vi "Read Coils.vi"(8 "error in (no error)":errorcluster, 9 "quantity":u16, 10 "starting address":u16, 11 "MB session in":refnum<class "MB_Master.lvclass">) -> (0 "error out":errorcluster, 2 "Coils":bool[](array[boolean]), 3 "MB session out":refnum<class "MB_Master.lvclass">)   [LabVIEW 2021, in "MB Master.lvlib"]
doc: "Function Code 1: Reads <b>quantity</b> number of coils starting from <b>starting address</b>"
uses:
  <vilib>/Plasmionique/MB Master/MB Master.lvlib
  <vilib>/Plasmionique/MB Master/MB_Master/MB_Master.lvclass
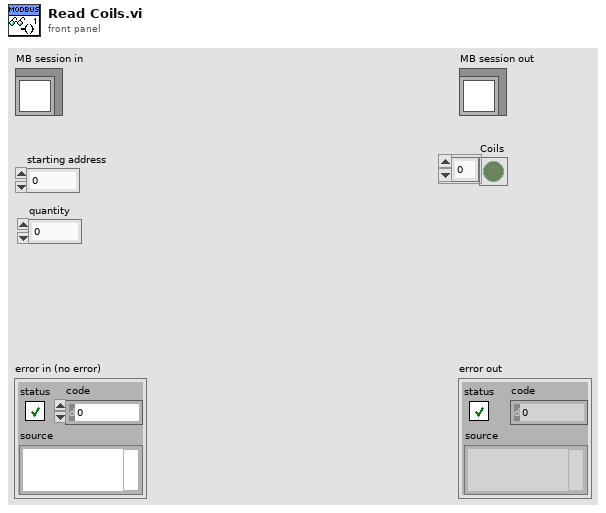
[diagram p1: front panel]
types:
  T1 = typedef "MB Master.lvlib/MB_PDU_Cluster.ctl" = cluster{"Function Code":u8, "Data":u8[], "RTU_DataBytes":i32}
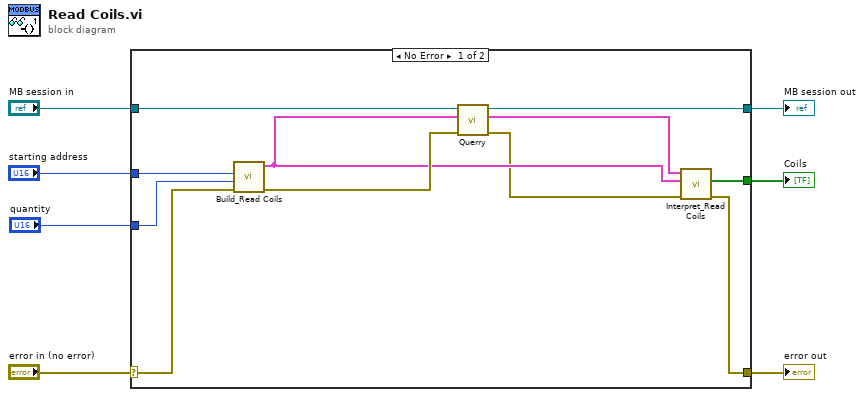
[diagram p0: block diagram]
diagram:
  n1 = case shown="No Error" "error in (no error)" {
    selector: "error in (no error)" -> [w15 w20]
    tunnel: [w8 w20] -> w6
    tunnel: [w13 w19] -> w4
    tunnel: "MB session in" -> [w14 w19]
    tunnel: "starting address" -> [w18 _]
    tunnel: "quantity" -> [w17 _]
    tunnel: [w10 _] -> w1
    frame No Error {
      n2 = call <vilib>:"Build_Read Coils.vi"("error in (no error)"=w15, "quantity"=w17, "starting address"=w18) -> ("error out"=w16:errorcluster, "MB_PDU"=w11:T1)  [unwired: 7 in]
      n3 = call-dynamic "Querry.vi"("error in (no error)"=w16, "PDU_req"=w11, "MB_Master in"=w14) -> ("error out"=w9:errorcluster, "PDU_resp"=w12:T1, "MB_Master out"=w13:refnum<class "MB_Master.lvclass">)  [unwired: 6 in]
      n4 = call <vilib>:"Interpret_Read Coils.vi"("error in (no error)"=w9, "MB_PDU_req in"=w11, "MB_PDU_resp in"=w12) -> ("error out"=w8:errorcluster, "Coils"=w10:bool[])  [unwired: 7 in]
    }
    frame Error {
    }
  }
  "error out" <- w6
  "MB session out" <- w4
  "Coils" <- w1
